vi "UI Interlocks.vi"(7 "Menu Ref":refnum<k9>, 8 "error in (no error)":errorcluster, 9 "Saved Macro":refnum<class "Macro.lvclass">, 10 "New Macro":refnum<class "Macro.lvclass">, 11 "Refs":T1) -> (0 "error out":errorcluster)   [LabVIEW 2020, in "MacroAssert.lvlib"]
doc: "Enables and disables controls based on the current state of the interface."
uses:
  MacroAssert.lvlib
  Classes/Macro/Macro.lvclass
  Classes/Step/Step.lvclass
  <userlib>/_MGI/Application Control/MGI Gray if/MGI Gray if False.vi
  CTLs/Refs.ctl
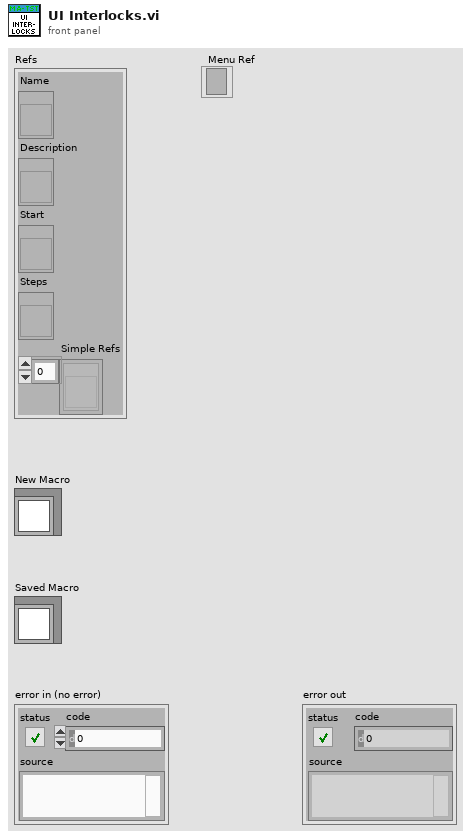
[diagram p1: front panel]
types:
  T1 = typedef "MacroAssert.lvlib/Refs.ctl" = cluster{"Name":refnum<vi>, "Description":refnum<vi>, "Start":refnum<vi>, "Steps":refnum<vi>, "Simple Refs":refnum<vi>[]}
  T2 = enum8{"Enabled", "Disabled", "Disabled and Grayed Out"}
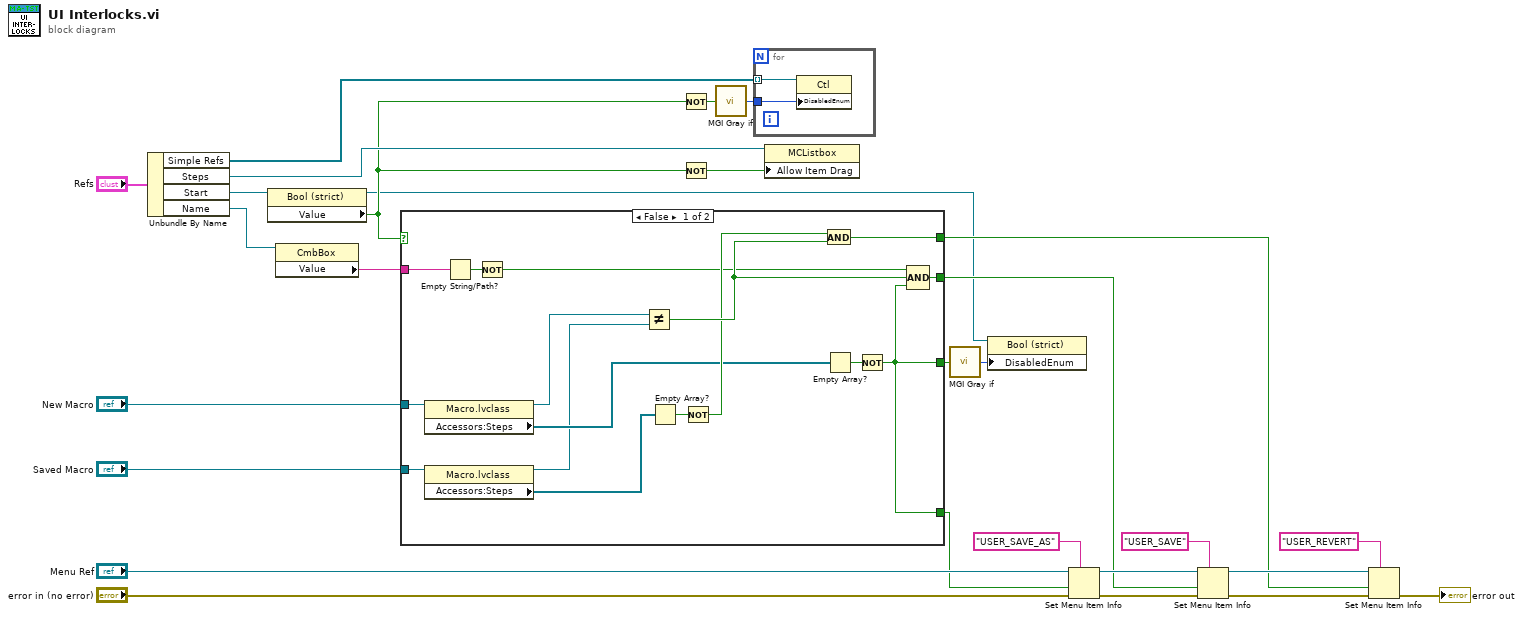
[diagram p0: block diagram]
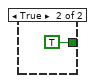
[diagram p2: hidden frame]
diagram:
  n1 = Unbundle By Name("Refs") -> ("Simple Refs"=w20:refnum<vi>[], "Steps"=w25:refnum<vi>, "Start"=w21:refnum<vi>, "Name"=w2:refnum<vi>)
  n2 = property class="Bool (strict)"(reference=w21) -> (reference out=w3:refnum<vi>, "Value"=w17:bool)  [unwired: 1 in, 1 out]
  n3 = property class="CmbBox"(reference=w2) -> ("Value"=w1:string)  [unwired: 1 in, 2 out]
  n4 = case shown="False" w17 {
    tunnel: [w42 _] -> w8
    tunnel: [w37 TRUE] -> w24
    tunnel: [w38 _] -> w4
    tunnel: [w37 _] -> w9
    tunnel: "New Macro" -> [w36 _]
    tunnel: "Saved Macro" -> [w35 _]
    tunnel: w1 -> [w30 _]
    frame False {
      n5 = property class="Macro.lvclass"(reference=w36) -> (reference out=w32:refnum<class "Macro.lvclass">, "Accessors:Steps"=w33:refnum<class "Step.lvclass">[])  [unwired: 1 in, 1 out]
      n6 = property class="Macro.lvclass"(reference=w35) -> (reference out=w31:refnum<class "Macro.lvclass">, "Accessors:Steps"=w34:refnum<class "Step.lvclass">[])  [unwired: 1 in, 1 out]
      n7 = Empty String/Path?(string/path=w30) -> (empty?=w43:bool)
      n8 = Not(x=w43) -> (.not. x?=w29:bool)
      n9 = Not Equal?(x=w32, y=w31) -> (x != y?=w40:bool)
      n10 = Empty Array?(array=w34) -> (empty?=w41:bool)
      n11 = Not(x=w41) -> (.not. x?=w39:bool)
      n12 = And(x=w39, y=w40) -> (x .and. y?=w38:bool)
      n13 = Empty Array?(array=w33) -> (empty?=w44:bool)
      n14 = Not(x=w44) -> (.not. x?=w37:bool)
      n15 = Compound Arithmetic op=AND(w29, w40, w37) -> (w42:bool)
    }
    frame True {
    }
  }
  n16 = Not(x=w17) -> (.not. x?=w18:bool)
  n17 = Not(x=w17) -> (.not. x?=w16:bool)
  n18 = call-poly <userlib>:"MGI Gray if.vi"("Boolean"=w18) -> ("Disabled"=w19:T2)
  n19 = for {
    tunnel: w20 -> [w47] mode=indexing
    tunnel: w19 -> [w46]
    n20 = property class="Ctl"(reference=w47, "DisabledEnum"=w46) -> ()  [unwired: 1 in, 2 out]
  }
  n21 = property class="MCListbox"(reference=w25, "Allow Item Drag"=w16) -> ()  [unwired: 1 in, 2 out]
  n22 = call-poly <userlib>:"MGI Gray if.vi"("Boolean"=w24) -> ("Disabled"=w23:T2)
  n23 = property on="Property Node" class="Bool (strict)"(reference=w3, "DisabledEnum"=w23) -> ()  [unwired: 1 in, 2 out]
  n24 = Set Menu Item Info(7:"USER_SAVE_AS" ("item tag"), 8:"error in (no error)", 9:w9, 11:"Menu Ref") -> (0:w10:errorcluster, 3:w27:refnum<k9>)  [unwired: 3 in]
  n25 = Set Menu Item Info(7:"USER_SAVE" ("item tag"), 8:w10, 9:w8, 11:w27) -> (0:w6:errorcluster, 3:w26:refnum<k9>)  [unwired: 3 in]
  n26 = Set Menu Item Info(7:"USER_REVERT" ("item tag"), 8:w6, 9:w4, 11:w26) -> (0:→"error out":errorcluster)  [unwired: 3 in, 1 out]
